vi "No callers--constant.vi"() -> (3 "No callers":string)   [LabVIEW 2021, in "TAF Proj Document Type.lvlib"]
uses:
  <vilib>/Wovalab/AntiDoc/Document Type/Add-ons/LabVIEW TAF Project/TAF Proj Document Type.lvlib
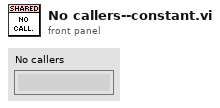
[diagram p1: front panel]
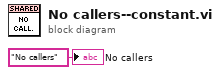
[diagram p0: block diagram]
diagram:
  "No callers" <- "No callers" ("Empty Description")
